vi "Button Reference.vi"(7 "Ref In":refnum<vi>, 11 "Command":string) -> (3 "Ref Out":refnum<vi>)   [LabVIEW 2015]
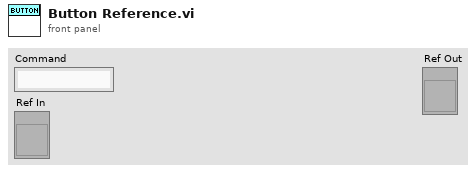
[diagram p1: front panel]
types:
  T1 = enum8{"Enabled", "Disabled", "Disabled and Grayed Out"}
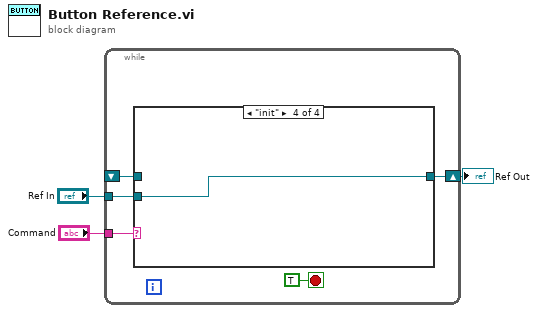
[diagram p0: block diagram]
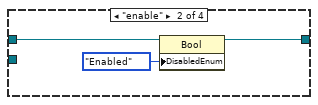
[diagram p3: hidden frame]
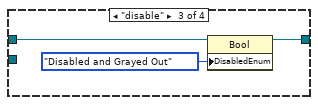
[diagram p4: hidden frame]
diagram:
  n1 = while {
    tunnel: "Command" -> [w7]
    shift-right: [w5] -> w3
    shift-left: _ -> [w6]
    tunnel: "Ref In" -> [w4]
    stop <- TRUE stop-if-true
    n2 = case shown="\"init\"" w7 {
      tunnel: w6 -> [w9 w12 w15 _]
      tunnel: [w9 w10 w13 w16] -> w5
      tunnel: w4 -> [_ _ _ w16]
      frame "read", Default {
      }
      frame "enable" {
        n3 = property class="Bool"(reference=w12, "DisabledEnum"=T1."Enabled" ("Disabled")) -> (reference out=w10:refnum<vi>)  [unwired: 1 in, 1 out]
      }
      frame "disable" {
        n4 = property class="Bool"(reference=w15, "DisabledEnum"=T1."Disabled and Grayed Out" ("Disabled")) -> (reference out=w13:refnum<vi>)  [unwired: 1 in, 1 out]
      }
      frame "init" {
      }
    }
  }
  "Ref Out" <- w3
